vi "FancyDrive.vi"(8 "Y axis value":dbl, 11 "X axis value":dbl) -> (0 "Right Motor Value":dbl, 3 "Left Motor Value":dbl)   [LabVIEW 2020]
uses:
  <vilib>/Rock Robotics/WPI/Joystick/WPI_JoystickArcadeMapping.vi
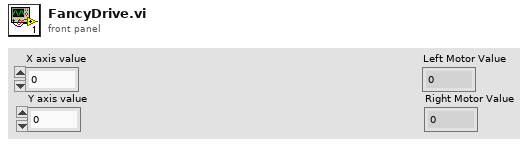
[diagram p1: front panel]
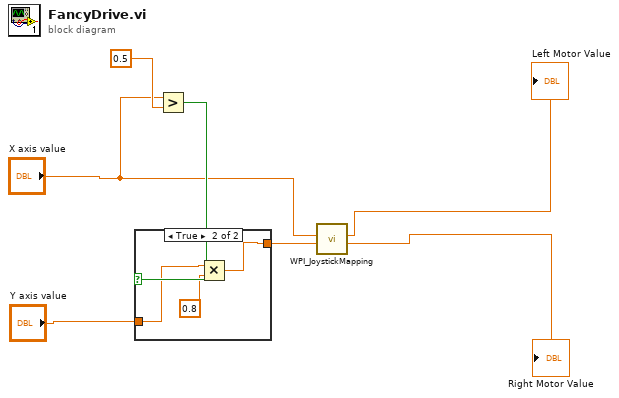
[diagram p0: block diagram]
diagram:
  n1 = Greater?(x="X axis value", y=0.5) -> (0:w4:bool)
  n2 = case shown="True" w4 {
    tunnel: [w8 w9] -> w3
    tunnel: "Y axis value" -> [w8 w10]
    frame False {
    }
    frame True {
      n3 = Multiply(x=w10, y=0.8) -> (x*y=w9:dbl)
    }
  }
  n4 = call-poly <vilib>:"WPI_JoystickMapping.vi"("Y axis value"=w3, "X axis value"="X axis value") -> ("Right Motor Value"=→"Right Motor Value":dbl, "Left Motor Value"=→"Left Motor Value":dbl)  [unwired: 8 in]
